vi "Proper Deadband.vi"(1 "Value":dbl) -> (0 "Deadbanded Value":dbl)   [LabVIEW 2011]
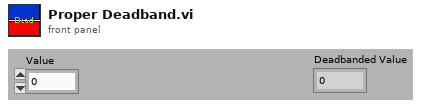
[diagram p1: front panel]
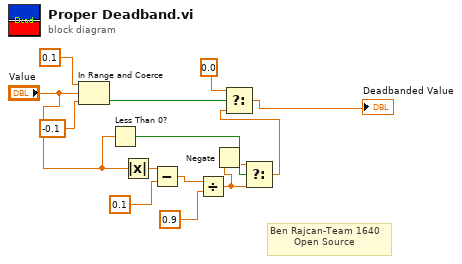
[diagram p0: block diagram]
diagram:
  # "Ben Rajcan-Team 1640\n        Open Source"
  n1 = In Range and Coerce(upper limit=0.1, x="Value", lower limit=-0.1) -> (In Range?=w12:bool)  [unwired: 1 out]
  n2 = Less Than 0?(x="Value") -> (x < 0?=w6:bool)
  n3 = Absolute Value(x="Value") -> (abs(x)=w10:dbl)
  n4 = Subtract(x=w10, y=0.1) -> (x-y=w8:dbl)
  n5 = Divide(x=w8, y=0.9) -> (x/y=w4:dbl)
  n6 = Negate(x=w4) -> (-x=w5:dbl)
  n7 = Select(t=w5, s=w6, f=w4) -> (s? t:f=w2:dbl)
  n8 = Select(t=0.0, s=w12, f=w2) -> (s? t:f=→"Deadbanded Value":dbl)
